vi "Visible Optics.VI"() -> ()   [LabVIEW 2020]
panel:
  in  "Case Constant\n(See Context Help)":bool
  in  "Loading State":T1(ring)=enum."Load Globals"
  in  "stop":bool
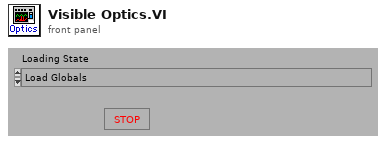
[diagram p1: front panel]
types:
  T1 = enum16{"--Quit--", "Load Globals", "Load Master", "Load Spectrometer", "Load Field", "Load Temperature", "Load Misc"}
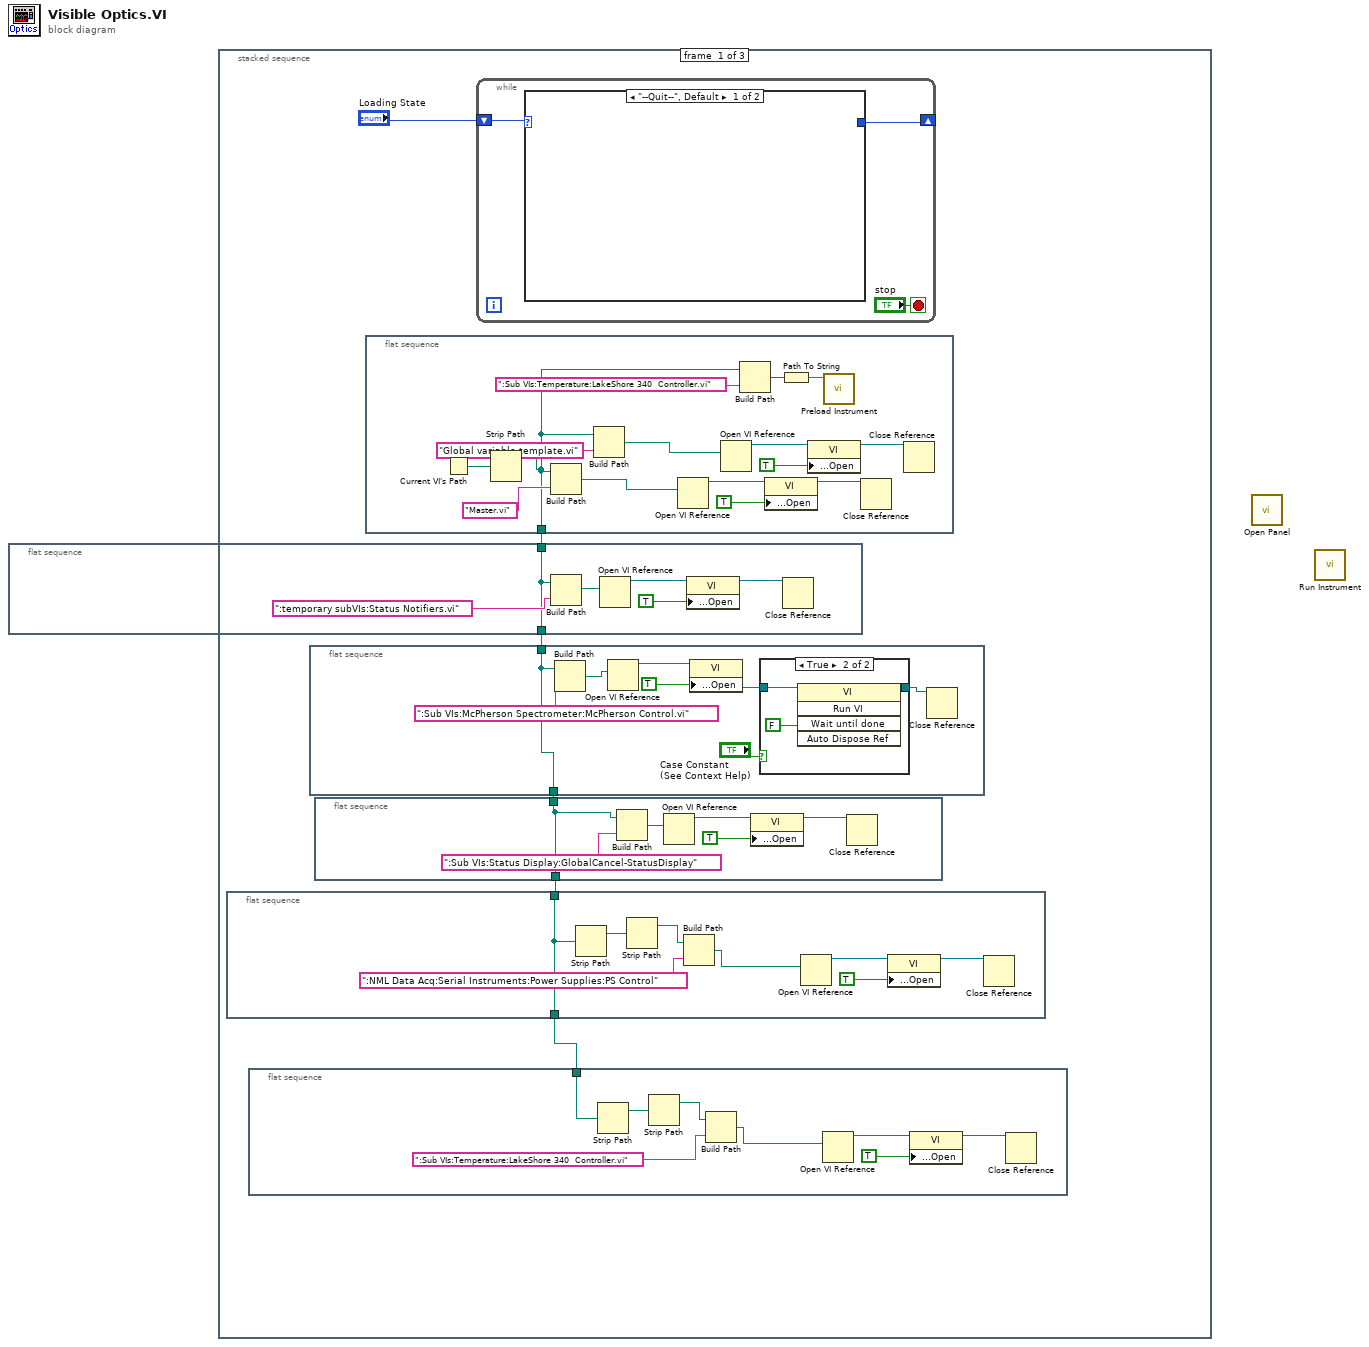
[diagram p0: block diagram]
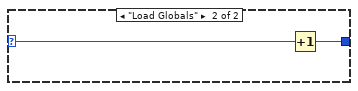
[diagram p2: hidden frame]
diagram:
  n1 = stacked-sequence {
    frame #0 {
      n2 = flat-sequence {
        tunnel: w6 -> [w46]
        tunnel: [w46] -> w5
        frame #0 {
          n3 = Build Path(base path=w46, name or relative path=":temporary subVIs:Status Notifiers.vi") -> (appended path=w47:path)
          n4 = Open VI Reference(vi path=w47) -> (vi reference=w50:refnum<vi>)  [unwired: 5 in, 1 out]
          n5 = property class="VI"(reference=w50, "Front Panel Window:Open"=TRUE) -> (reference out=w51:refnum<vi>)  [unwired: 1 in, 1 out]
          n6 = Close Reference(reference=w51) -> ()  [unwired: 1 in, 1 out]
        }
      }
      n7 = flat-sequence {
        tunnel: w3 -> [w26]
        tunnel: [w26] -> w2
        frame #0 {
          n8 = Strip Path(path=w26) -> (stripped path=w30:path)  [unwired: 1 out]
          n9 = Strip Path(path=w30) -> (stripped path=w29:path)  [unwired: 1 out]
          n10 = Build Path(base path=w29, name or relative path=":NML Data Acq:Serial Instruments:Power Supplies:PS Control") -> (appended path=w27:path)
          n11 = Open VI Reference(vi path=w27) -> (vi reference=w32:refnum<vi>)  [unwired: 5 in, 1 out]
          n12 = property class="VI"(reference=w32, "Front Panel Window:Open"=TRUE) -> (reference out=w33:refnum<vi>)  [unwired: 1 in, 1 out]
          n13 = Close Reference(reference=w33) -> ()  [unwired: 1 in, 1 out]
        }
      }
      n14 = flat-sequence {
        tunnel: w2 -> [w16]
        frame #0 {
          n15 = Strip Path(path=w16) -> (stripped path=w15:path)  [unwired: 1 out]
          n16 = Strip Path(path=w15) -> (stripped path=w14:path)  [unwired: 1 out]
          n17 = Build Path(base path=w14, name or relative path=":Sub VIs:Temperature:LakeShore 340  Controller.vi") -> (appended path=w12:path)
          n18 = Open VI Reference(vi path=w12) -> (vi reference=w18:refnum<vi>)  [unwired: 5 in, 1 out]
          n19 = property class="VI"(reference=w18, "Front Panel Window:Open"=TRUE) -> (reference out=w19:refnum<vi>)  [unwired: 1 in, 1 out]
          n20 = Close Reference(reference=w19) -> ()  [unwired: 1 in, 1 out]
        }
      }
      n21 = flat-sequence {
        tunnel: w5 -> [w34]
        tunnel: [w34] -> w4
        frame #0 {
          n22 = Build Path(base path=w34, name or relative path=":Sub VIs:McPherson Spectrometer:McPherson Control.vi") -> (appended path=w37:path)
          n23 = Open VI Reference(vi path=w37) -> (vi reference=w39:refnum<vi>)  [unwired: 5 in, 1 out]
          n24 = property class="VI"(reference=w39, "Front Panel Window:Open"=TRUE) -> (reference out=w40:refnum<vi>)  [unwired: 1 in, 1 out]
          n25 = case shown="True" "Case Constant\n(See Context Help)" {
            tunnel: [w42 w44] -> w41
            tunnel: w40 -> [w42 w43]
            frame False {
            }
            frame True {
              n26 = invoke class="VI" method="Run VI"(reference=w43, "Wait until done"=FALSE ("Execution:Run When Opened")) -> (reference out=w44:refnum<vi>)  [unwired: 3 in, 4 out]
            }
          }
          n27 = Close Reference(reference=w41) -> ()  [unwired: 1 in, 1 out]
        }
      }
      n28 = flat-sequence {
        tunnel: w4 -> [w20]
        tunnel: [w20] -> w3
        frame #0 {
          n29 = Build Path(base path=w20, name or relative path=":Sub VIs:Status Display:GlobalCancel-StatusDisplay") -> (appended path=w22:path)
          n30 = Open VI Reference(vi path=w22) -> (vi reference=w24:refnum<vi>)  [unwired: 5 in, 1 out]
          n31 = property class="VI"(reference=w24, "Front Panel Window:Open"=TRUE) -> (reference out=w25:refnum<vi>)  [unwired: 1 in, 1 out]
          n32 = Close Reference(reference=w25) -> ()  [unwired: 1 in, 1 out]
        }
      }
      n33 = flat-sequence {
        tunnel: [w55] -> w6
        frame #0 {
          n34 = Current VI's Path() -> (path=w63:path)
          n35 = Strip Path(path=w63) -> (stripped path=w55:path)  [unwired: 1 out]
          n36 = Build Path(base path=w55, name or relative path="Master.vi") -> (appended path=w61:path)
          n37 = Build Path(base path=w55, name or relative path="Global variable template.vi") -> (appended path=w57:path)
          n38 = Open VI Reference(vi path=w61) -> (vi reference=w65:refnum<vi>)  [unwired: 5 in, 1 out]
          n39 = Open VI Reference(vi path=w57) -> (vi reference=w59:refnum<vi>)  [unwired: 5 in, 1 out]
          n40 = Build Path(base path=w55, name or relative path=":Sub VIs:Temperature:LakeShore 340  Controller.vi") -> (appended path=w53:path)
          n41 = property class="VI"(reference=w65, "Front Panel Window:Open"=TRUE) -> (reference out=w66:refnum<vi>)  [unwired: 1 in, 1 out]
          n42 = Path To String(path=w53) -> (string=w52:string)
          n43 = property class="VI"(reference=w59, "Front Panel Window:Open"=TRUE) -> (reference out=w60:refnum<vi>)  [unwired: 1 in, 1 out]
          n44 = call <vilib>:"Preload Instrument.vi"("VI name"=w52) -> ()  [unwired: 10 in, 1 out]
          n45 = Close Reference(reference=w66) -> ()  [unwired: 1 in, 1 out]
          n46 = Close Reference(reference=w60) -> ()  [unwired: 1 in, 1 out]
        }
      }
      n47 = while {
        shift-right: [w7] -> _
        shift-left: "Loading State" -> [w8]
        stop <- "stop" stop-if-true
        n48 = case shown="\"--Quit--\", Default" w8 {
          selector: w8 -> [_ w10]
          tunnel: [_ w11] -> w7
          frame "--Quit--", Default {
          }
          frame "Load Globals" {
            n49 = Increment(x=w10) -> (x+1=w11:T1)
          }
        }
      }
    }
    frame #1 {
    }
    frame #2 {
    }
  }
  n50 = call <vilib>:"Open Panel.vi"() -> ()  [unwired: 11 in, 1 out]
  n51 = call <vilib>:"Run Instrument.vi"() -> ()  [unwired: 11 in, 1 out]
